vi "DSF.Engine.Hardware Info.Set CPU.vi"(8 "error in (no error)":errorcluster, 10 "CPU Info":refnum<class "DSF.Engine.Hardware Info.CPU.lvclass">, 11 "Hardware Info in":refnum<class "DSF.Engine.Hardware Info.lvclass">) -> (0 "error out":errorcluster, 3 "Hardware Info out":refnum<class "DSF.Engine.Hardware Info.lvclass">)   [LabVIEW 2017, in "DSF.Engine.lvlib" / "DSF.Engine.Hardware Info.lvclass"]
uses:
  DSF.Engine.Hardware Info.lvclass
  DSF.Engine.Hardware Info.CPU.lvclass
  DSF.Engine.Hardware Info.lvclass/DSF.Engine.Hardware Info.ctl
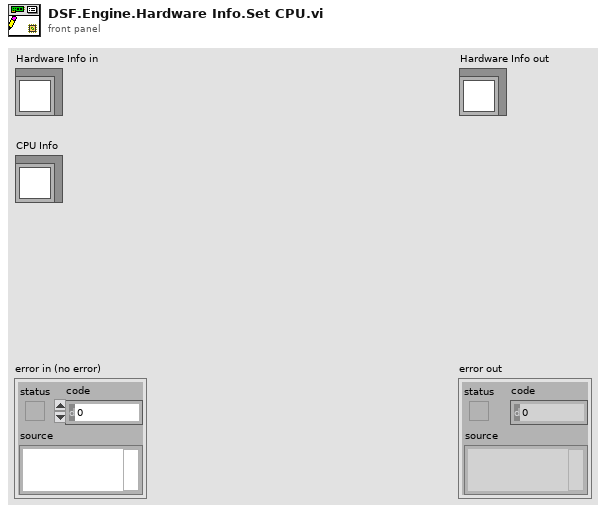
[diagram p1: front panel]
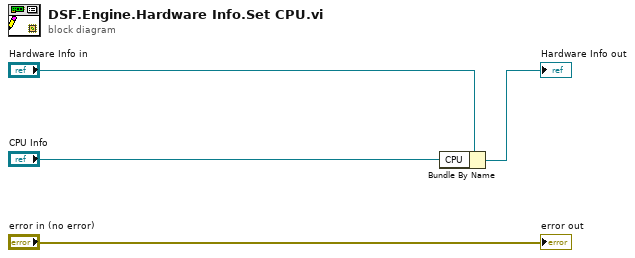
[diagram p0: block diagram]
diagram:
  n1 = Bundle By Name(cluster="Hardware Info in", "CPU"="CPU Info") -> (→"Hardware Info out":refnum<class "DSF.Engine.Hardware Info.lvclass">)
  "error out" <- "error in (no error)"
